vi "AddRequestCreate.vi"(9 "New Name":string, 10 "TypeDefPath":path, 11 "VI in":refnum<vi>) -> (0 "error out":errorcluster)   [LabVIEW 2024, in "AddNewEvent.lvlib"]
uses:
  Event/AddNewEvent.lvlib
  <vilib>/Utility/traverseref.llb/TRef TravTarget.ctl
  Event/Templates/RequestRegTemplate.vi
  <vilib>/Utility/traverseref.llb/VI Scripting - Traverse.lvlib
panel:
  out "# of Refs":i32
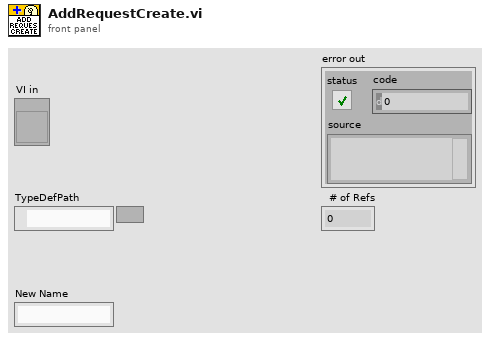
[diagram p1: front panel]
types:
  T1 = typedef "TRef TravTarget.ctl" = enum16{"FP", "BD", "Other"}
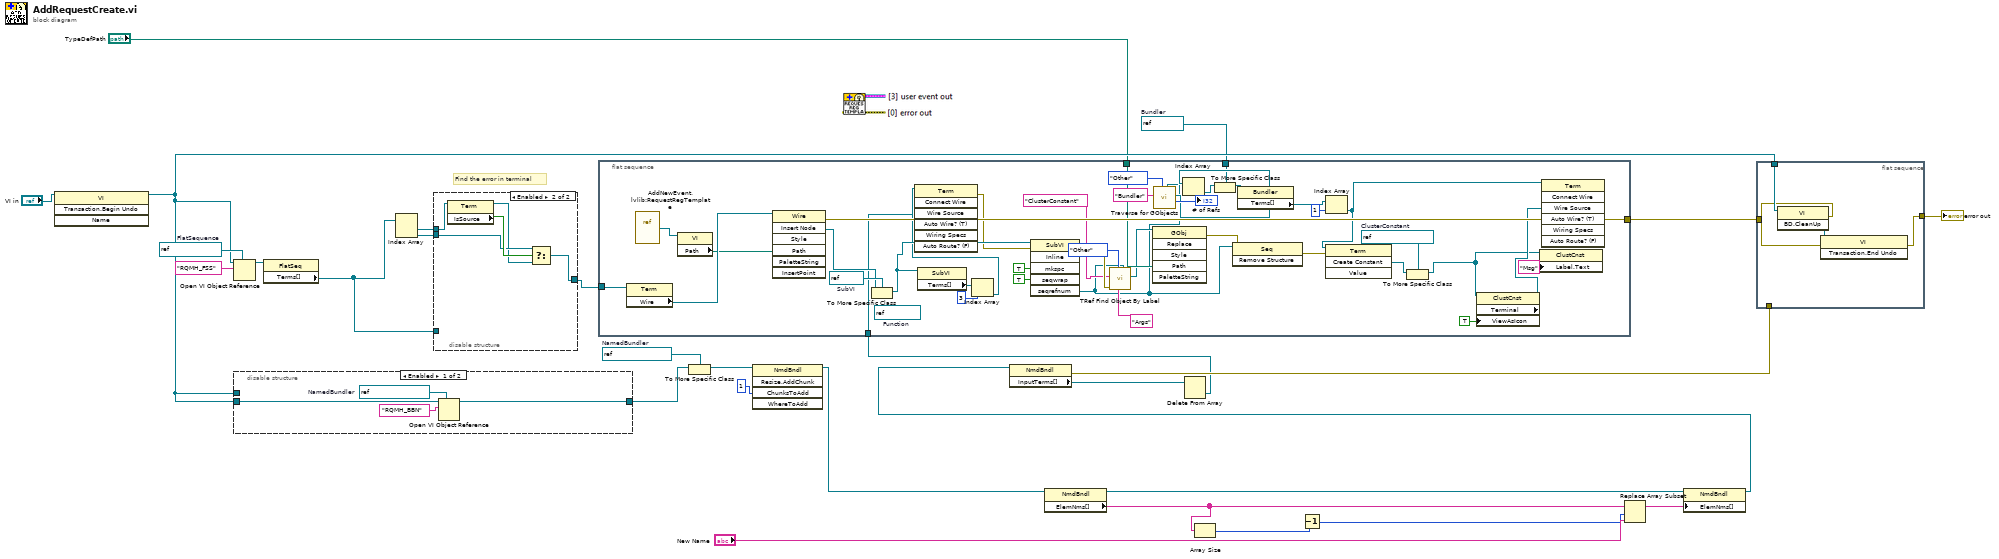
[diagram p0: block diagram]
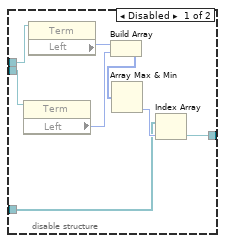
[diagram p2: hidden frame]
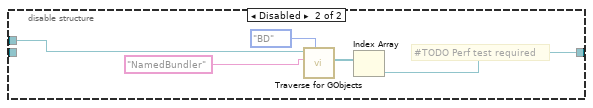
[diagram p3: hidden frame]
diagram:
  w1 = refnum<vi> refnum  # Bundler
  w26 = refnum<vi> refnum  # FlatSequence
  w22 = refnum<vi> refnum  # NamedBundler
  # "Find the error in terminal"
  n1 = invoke class="VI" method="Transaction.Begin Undo"(reference="VI in") -> (reference out=w6:refnum<vi>)  [unwired: 3 in, 3 out]
  n2 = Open VI Object Reference(7:w26, 10:"RQMH_FSS" ("name/order"), 11:w6) -> (3:w28:refnum<vi>)  [unwired: 1 in, 1 out]
  n3 = disable-structure shown="Enabled" {
    disable-tunnel: w6 -> [w31 _]
    disable-tunnel: w6 -> [_ w34]
    disable-tunnel: [w29 w33] -> w27
    frame Enabled {
      w30 = refnum<vi> refnum  # NamedBundler
      n4 = Open VI Object Reference(7:w30, 10:"RQMH_BBN" ("name/order"), 11:w31) -> (3:w29:refnum<vi>)  [unwired: 1 in, 1 out]
    }
    frame Disabled {
      # "#TODO Perf test required"
      n5 = call <vilib>:"Traverse for GObjects.vi"("Traverse Target"=TRef_TravTarget."BD", "Class Name"="NamedBundler", "VI Refnum"=w34) -> ("References"=w37:refnum<vi>[])  [unwired: 5 in, 3 out]
      n6 = Index Array(array=w37) -> (element=w33:refnum<vi>)  [unwired: 1 in]
    }
  }
  n7 = property class="FlatSeq"(reference=w28) -> ("Terms[]"=w10:refnum<vi>[])  [unwired: 1 in, 2 out]
  n8 = Index Array(array=w10) -> (element #1=w11:refnum<vi>, element #2=w12:refnum<vi>)  [unwired: 2 in]
  n9 = disable-structure shown="Enabled" {
    disable-tunnel: w12 -> [w41 w47]
    disable-tunnel: w11 -> [w40 w50]
    disable-tunnel: w10 -> [w39 _]
    disable-tunnel: [w38 w48] -> w9
    frame Disabled {
      n10 = property class="Term"(reference=w41) -> ("Left"=w43:i32)  [unwired: 1 in, 2 out]
      n11 = property class="Term"(reference=w40) -> ("Left"=w42:i32)  [unwired: 1 in, 2 out]
      n12 = Build Array(w42, w43) -> (w44:i32[])
      n13 = Array Max & Min(array=w44) -> (min index (indices)=w45:i32)  [unwired: 3 out]
      n14 = Index Array(array=w39, index=w45) -> (element=w38:refnum<vi>)
    }
    frame Enabled {
      n15 = property class="Term"(reference=w50) -> (reference out=w46:refnum<vi>, "IsSource"=w49:bool)  [unwired: 1 in, 1 out]
      n16 = Select(t=w47, s=w49, f=w46) -> (s? t:f=w48:refnum<vi>)
    }
  }
  n17 = flat-sequence {
    tunnel: w9 -> [w90]
    tunnel: [w86] -> w5
    tunnel: "TypeDefPath" -> [w81]
    tunnel: w2 -> [w67]
    tunnel: w1 -> [w62]
    frame #0 {
      w52 = refnum<vi> refnum  # ClusterConstant
      (unwired) refnum<vi> refnum  # Function
      w85 = refnum<vi> refnum  # SubVI
      n18 = property class="Term"(reference=w90) -> ("Wire"=w89:refnum<vi>)  [unwired: 1 in, 2 out]
      n19 = vi-ref "AddNewEvent.lvlib:RequestRegTemplate.vi"() -> (w88:refnum<vi>)
      n20 = property class="VI"(reference=w88) -> ("Path"=w87:path)  [unwired: 1 in, 2 out]
      n21 = invoke class="Wire" method="Insert Node"(reference=w89, "Path"=w87) -> (error out=w86:errorcluster, "Insert Node"=w84:refnum<vi>)  [unwired: 5 in, 5 out]
      n22 = To More Specific Class(target class=w85, reference=w84) -> (specific class reference=w71:refnum<vi>)  [unwired: 1 in, 1 out]
      n23 = property class="SubVI"(reference=w71) -> ("Terms[]"=w70:refnum<vi>[])  [unwired: 1 in, 2 out]
      n24 = Index Array(array=w70, index=3) -> (element=w68:refnum<vi>)
      n25 = invoke class="Term" method="Connect Wire"(reference=w68, "Wire Source"=w67) -> (error out=w58:errorcluster)  [unwired: 5 in, 6 out]
      n26 = invoke class="SubVI" method="Inline"(reference=w71, error in=w58, "mkspc"=TRUE ("Make Space in Block Diagram"), "seqwrap"=TRUE ("Wrap in Sequence")) -> (error out=w79:errorcluster, "seqrefnum"=w63:refnum<vi>)  [unwired: 2 in, 4 out]
      n27 = call <vilib>:"TRef Find Object By Label.vi"("Other Refnum"=w63, "Label"="Args" ("name/order"), "Traverse Target"=TRef_TravTarget."Other", "error in (no error)"=w79, "Class Name"="ClusterConstant" ("name/order")) -> ("Found Obj Ref"=w75:refnum<vi>)  [unwired: 3 in, 3 out]
      n28 = invoke class="GObj" method="Replace"(reference=w75, "Path"=w81) -> (error out=w80:errorcluster)  [unwired: 4 in, 5 out]
      n29 = call <vilib>:"Traverse for GObjects.vi"("Other Refnum"=w63, "Traverse Target"=TRef_TravTarget."Other", "Class Name"="Bundler") -> ("# of Refs"=→"# of Refs":i32, "References"=w66:refnum<vi>[])  [unwired: 5 in, 2 out]
      n30 = Index Array(array=w66) -> (element=w65:refnum<vi>)  [unwired: 1 in]
      n31 = To More Specific Class(target class=w62, reference=w65) -> (specific class reference=w64:refnum<vi>)  [unwired: 1 in, 1 out]
      n32 = invoke class="Seq" method="Remove Structure"(reference=w63, error in=w80) -> (error out=w60:errorcluster)  [unwired: 1 in, 2 out]
      n33 = property class="Bundler"(reference=w64) -> ("Terms[]"=w61:refnum<vi>[])  [unwired: 1 in, 2 out]
      n34 = Index Array(array=w61, index=1) -> (element=w57:refnum<vi>)
      n35 = invoke class="Term" method="Create Constant"(reference=w57, error in=w60) -> ("Create Constant"=w54:refnum<vi>)  [unwired: 2 in, 3 out]
      n36 = To More Specific Class(target class=w52, reference=w54) -> (specific class reference=w53:refnum<vi>)  [unwired: 1 in, 1 out]
      n37 = property class="ClustCnst"(reference=w53, "ViewAsIcon"=TRUE ("View As Icon")) -> ("Terminal"=w55:refnum<vi>)  [unwired: 1 in, 2 out]
      n38 = property class="ClustCnst"(reference=w53, "Label.Text"="Msg") -> ()  [unwired: 1 in, 2 out]
      n39 = invoke class="Term" method="Connect Wire"(reference=w57, "Wire Source"=w55) -> ()  [unwired: 5 in, 7 out]
    }
  }
  n40 = To More Specific Class(target class=w22, reference=w27) -> (specific class reference=w23:refnum<vi>)  [unwired: 1 in, 1 out]
  n41 = invoke class="NmdBndl" method="Resize.AddChunk"(reference=w23, "ChunksToAdd"=u8 1 ("Chunks To Add")) -> (reference out=w15:refnum<vi>)  [unwired: 3 in, 4 out]
  n42 = property class="NmdBndl"(reference=w15) -> (reference out=w21:refnum<vi>, "ElemNms[]"=w18:string[])  [unwired: 1 in, 1 out]
  n43 = Array Size(array=w18) -> (size(s)=w17:i32)
  n44 = Decrement(x=w17) -> (x-1=w16:i32)
  n45 = Replace Array Subset(array=w18, new element="New Name", index=w16) -> (w20:string[])
  n46 = property class="NmdBndl"(reference=w21, "ElemNms[]"=w20) -> (reference out=w14:refnum<vi>)  [unwired: 1 in, 1 out]
  n47 = property class="NmdBndl"(reference=w14) -> (error out=w4:errorcluster, "InputTerms[]"=w25:refnum<vi>[])  [unwired: 1 in, 1 out]
  n48 = Delete From Array(array=w25) -> (deleted portion=w2:refnum<vi>)  [unwired: 2 in, 1 out]
  n49 = flat-sequence {
    tunnel: w6 -> [w94]
    tunnel: [w92] -> w8
    tunnel: w5 -> [_]
    tunnel: w4 -> [_]
    frame #0 {
      n50 = invoke class="VI" method="BD.CleanUp"(reference=w94) -> (reference out=w91:refnum<vi>, error out=w93:errorcluster)  [unwired: 2 in, 1 out]
      n51 = invoke class="VI" method="Transaction.End Undo"(reference=w91, error in=w93) -> (error out=w92:errorcluster)  [unwired: 1 in, 2 out]
    }
  }
  "error out" <- w8
